vi "Parameter to encoder value - Copia.vi"(8 "error in (no error)":errorcluster, 9 "parameter":dbl, 11 "Motor in":refnum<class "Motor.lvclass">) -> (0 "error out":errorcluster, 1 "encoder value":dbl, 2 "valid":bool, 3 "Motor out":refnum<class "Motor.lvclass">)   [LabVIEW 2018, in "Motor.lvclass"]
uses:
  Motor.lvclass
  Motor.lvclass/Motor.ctl
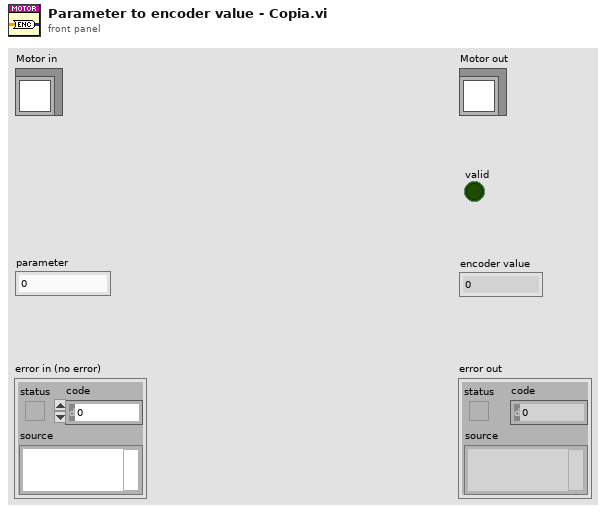
[diagram p1: front panel]
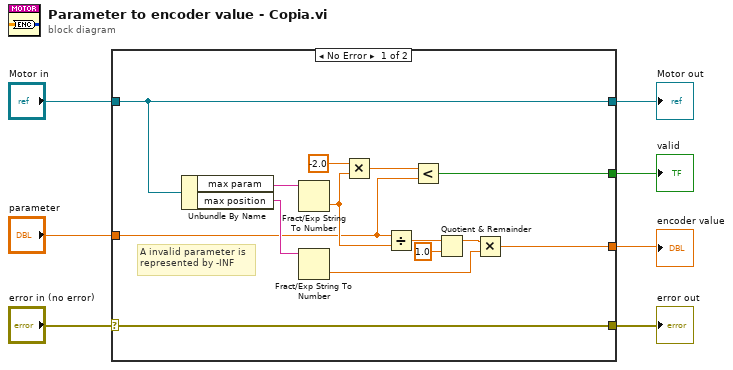
[diagram p0: block diagram]
diagram:
  n1 = case shown="No Error" "error in (no error)" {
    selector: "error in (no error)" -> [w21 w22]
    tunnel: [w21 w22] -> w6
    tunnel: [w20 w23] -> w4
    tunnel: "Motor in" -> [w20 w23]
    tunnel: "parameter" -> [w10 _]
    tunnel: [w9 _] -> w2
    tunnel: [w8 _] -> w1
    frame No Error {
      # "A invalid parameter is\nrepresented by -INF"
      n2 = Unbundle By Name(w20) -> ("max param"=w18:string, "max position"=w17:string)
      n3 = Fract/Exp String To Number(string=w18) -> (number=w13:dbl)  [unwired: 3 in, 1 out]
      n4 = Fract/Exp String To Number(string=w17) -> (number=w14:dbl)  [unwired: 3 in, 1 out]
      n5 = Multiply(x=-2.0, y=w13) -> (x*y=w11:dbl)
      n6 = Divide(x=w10, y=w13) -> (x/y=w19:dbl)
      n7 = Less?(x=w11, y=w10) -> (x < y?=w9:bool)
      n8 = Quotient & Remainder(x=w19, y=1.0) -> (x-y*floor(x/y)=w15:dbl)  [unwired: 1 out]
      n9 = Multiply(x=w15, y=w14) -> (x*y=w8:dbl)
    }
    frame Error {
    }
  }
  "error out" <- w6
  "Motor out" <- w4
  "valid" <- w2
  "encoder value" <- w1
